vi "lock-in reference global.vi"() -> ()   [LabVIEW 2015]
panel:
  out "data":waveform(dbl)
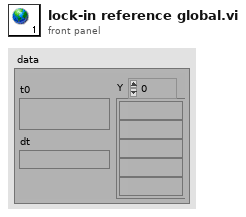
[diagram p1: front panel]
diagram:
